vi "Read Section Names.vi"(8 "error in (no error)":errorcluster, 11 "Interface in":refnum<class "Interface.lvclass">) -> (0 "error out":errorcluster, 1 "Section Names":string[](array[string]), 2 "Section Classes":path[](array[path]), 3 "Interface out":refnum<class "Interface.lvclass">)   [LabVIEW 2014, in "Configuration.lvlib" / "Interface.lvclass"]
doc: "Read available sections and pathes to corresponding derived class of Sections.lvclass."
uses:
  Interface.lvclass
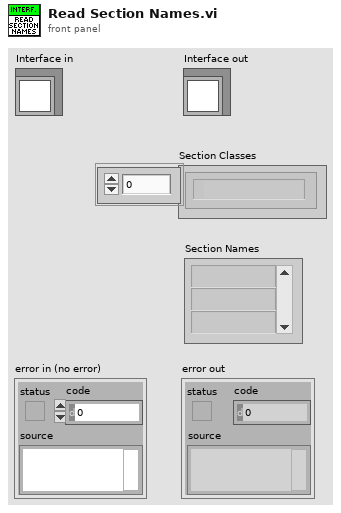
[diagram p1: front panel]
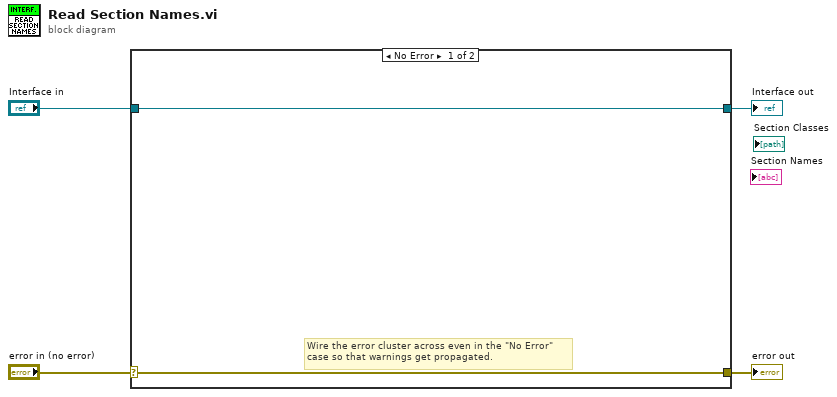
[diagram p0: block diagram]
diagram:
  n1 = case shown="No Error" "error in (no error)" {
    selector: "error in (no error)" -> [w5 w8]
    tunnel: [w5 w8] -> w3
    tunnel: [w6 w7] -> w1
    tunnel: "Interface in" -> [w6 w7]
    frame No Error {
      # "Wire the error cluster across even in the \"No Error\"\ncase so that warnings get propagated."
    }
    frame Error {
    }
  }
  "error out" <- w3
  "Interface out" <- w1
